vi "Greet World.vi"(7 "Hello (T)/Goodbye(F)":bool, 8 "error in (no error)":errorcluster, 11 "AbstractLanguage in":refnum<class "AbstractLanguage.lvclass">) -> (0 "error out":errorcluster, 2 "Grreting String":string, 3 "AbstractLanguage out":refnum<class "AbstractLanguage.lvclass">)   [LabVIEW 2019, in "AbstractLanguage.lvclass"]
uses:
  AbstractLanguage.lvclass
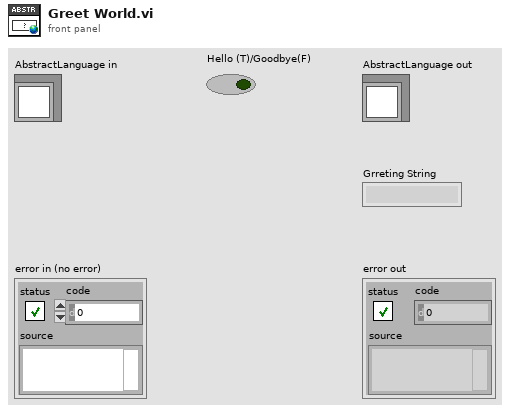
[diagram p1: front panel]
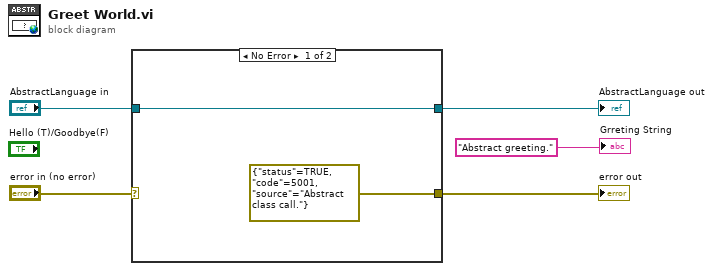
[diagram p0: block diagram]
diagram:
  n1 = case shown="No Error" "error in (no error)" {
    selector: "error in (no error)" -> [_ w9]
    tunnel: [errorcluster {"status"=TRUE, "code"=5001, "source"="Abstract class call."} ("error IO") w9] -> w4
    tunnel: [w7 w8] -> w2
    tunnel: "AbstractLanguage in" -> [w7 w8]
    frame No Error {
    }
    frame Error {
    }
  }
  "error out" <- w4
  "AbstractLanguage out" <- w2
  "Grreting String" <- "Abstract greeting." ("source")
